vi "add measure(SubVI).vi"(10 "字符串":string) -> (1 "ok or cancel":bool=TRUE, 2 "连接的字符串":string)   [LabVIEW 2019, in "Add Seq.lvlib"]
uses:
  Add Seq.lvlib
panel:
  in  "cancel":bool
  in  "ok":bool
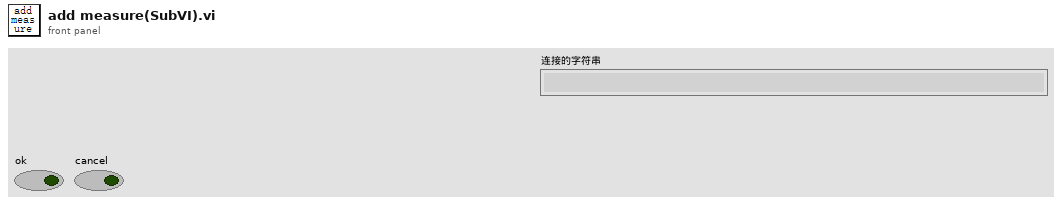
[diagram p1: front panel]
types:
  T1 = enum16{"open", "replace", "create", "open or create", "replace or create"}
  T2 = enum16{"open", "replace", "create", "open or create", "replace or create", "replace or create with confirmation"}
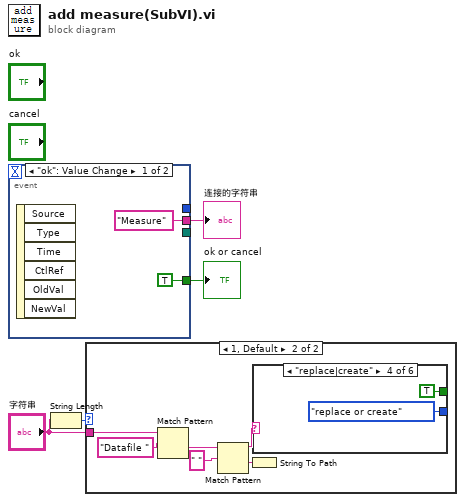
[diagram p0: block diagram]
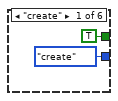
[diagram p3: hidden frame]
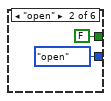
[diagram p4: hidden frame]
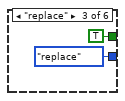
[diagram p5: hidden frame]
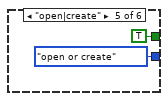
[diagram p6: hidden frame]
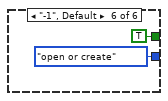
[diagram p7: hidden frame]
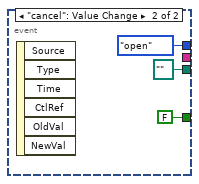
[diagram p8: hidden frame]
diagram:
  n1 = event shown="[0] \"ok\": Value Change" {
    selector: _ -> [_ _]
    dyn-events: _ -> [_ _]
    timeout: _ -> [_ _]
    tunnel: [_ path "" ("path")] -> _
    tunnel: [_ T1."open" ("operation(0:open)")] -> _
    tunnel: [TRUE FALSE] -> w4
    tunnel: ["Measure" ("连接的字符串") _] -> w1
    event "ok": Value Change {
      n2 = event-data() -> ()  [unwired: 1 in, 6 out]
    }
    event "cancel": Value Change {
      n3 = event-data() -> ()  [unwired: 1 in, 6 out]
    }
  }
  "连接的字符串" <- w1
  "ok or cancel" <- w4
  n4 = String Length(string="字符串") -> (length=w2:i32)
  n5 = case shown="1, Default" w2 {
    tunnel: "字符串" -> [_ w12]
    frame 0 {
    }
    frame 1, Default {
      n6 = Match Pattern(string=w12, regular expression="Datafile " ("正则表达式")) -> (after substring=w15:string)  [unwired: 1 in, 3 out]
      n7 = Match Pattern(string=w15, regular expression=" " ("正则表达式")) -> (before substring=w11:string, after substring=w13:string)  [unwired: 1 in, 2 out]
      n8 = String To Path(string=w13) -> ()  [unwired: 1 out]
      n9 = case shown="\"replace|create\"" w11 {
        tunnel: [T2."create" ("操作(0:open)") T2."open" ("操作(0:open)") T2."replace" ("操作(0:open)") T2."replace or create" ("操作(0:open)") T2."open or create" ("操作(0:open)") T2."open or create" ("操作(0:open)")] -> _
        tunnel: [TRUE FALSE TRUE TRUE TRUE TRUE] -> _
        frame "create" {
        }
        frame "open" {
        }
        frame "replace" {
        }
        frame "replace|create" {
        }
        frame "open|create" {
        }
        frame "-1", Default {
        }
      }
    }
  }
